vi "Create and configure UDL.vi"(8 "error in":errorcluster, 11 "file path (use dialog)":path) -> (0 "error out":errorcluster, 3 "UDL path":path)   [LabVIEW 2013, in "Database Lib.lvlib"]
uses:
  Database Lib.lvlib
panel:
  out "string":string
  out "cancelled":bool
  out "text":string
  # "Provider=;\nData Source=;\nMode=ReadWrite;\nPersist Security Info=False"
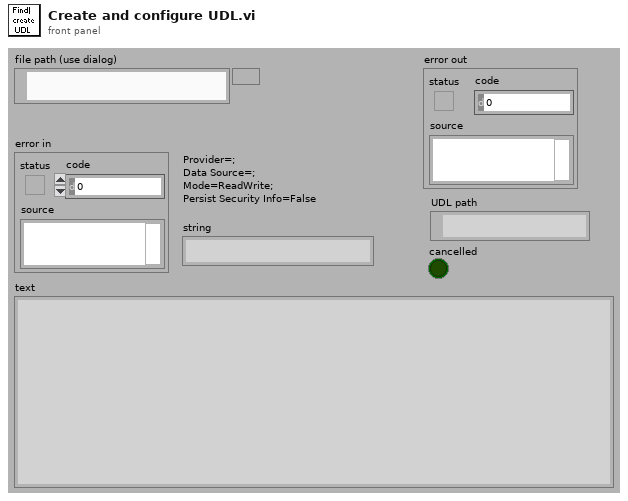
[diagram p1: front panel]
types:
  T1 = enum16{"open", "replace", "create", "open or create", "replace or create", "replace or create with confirmation"}
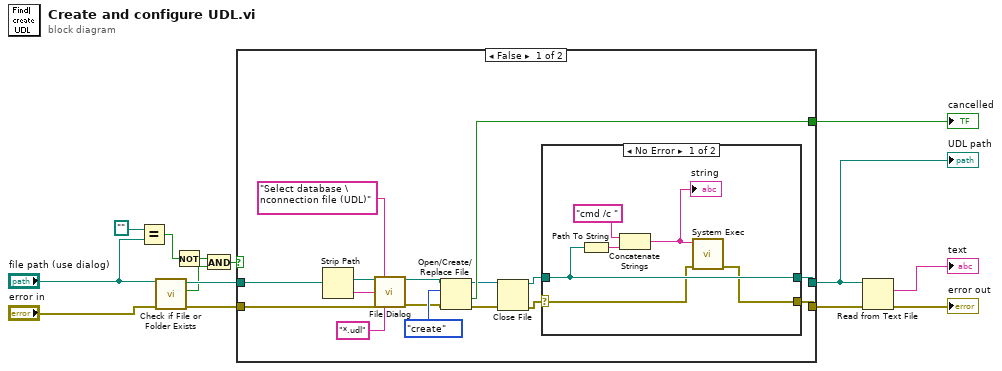
[diagram p0: block diagram]
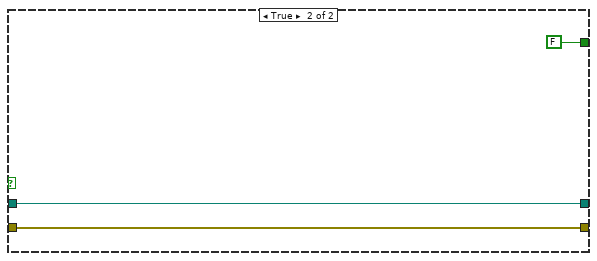
[diagram p3: hidden frame]
diagram:
  n1 = Equal?(x=path "", y="file path (use dialog)") -> (x = y?=w1:bool)
  n2 = call <vilib>:"Check if File or Folder Exists.vi"("error in (no error)"="error in", "path"="file path (use dialog)") -> ("error out"=w10:errorcluster, "file or folder exists?"=w5:bool, "dup path"=w11:path)  [unwired: 7 out]
  n3 = Not(x=w1) -> (.not. x?=w2:bool)
  n4 = And(x=w2, y=w5) -> (x .and. y?=w6:bool)
  n5 = case shown="False" w6 {
    tunnel: w11 -> [w15 w40]
    tunnel: w10 -> [w22 w41]
    tunnel: [w25 w41] -> w9
    tunnel: [w23 w40] -> w7
    tunnel: [w29 FALSE ("cancelled")] -> w8
    frame False {
      n6 = Strip Path(path=w15) -> (stripped path=w17:path, name=w16:string)
      n7 = call "File Dialog"("start path"=w17, "prompt"="Select database \nconnection file (UDL)", "default name"=w16, "error in"=w22, "pattern (all files)"="*.udl") -> ("selected path"=w20:path, "error out"=w21:errorcluster)  [unwired: 2 in, 7 out]
      n8 = Open/Create/Replace File(file path (use dialog)=w20, error in=w21, operation (0:open)=T1."create") -> (refnum out=w27:refnum<file>, cancelled=w29:bool, error out=w28:errorcluster)  [unwired: 3 out]
      n9 = Close File(refnum=w27, error in=w28) -> (path=w24:path, error out=w26:errorcluster)
      n10 = case shown="No Error" w26 {
        selector: w26 -> [w35 w38]
        tunnel: [w34 w38] -> w25
        tunnel: w24 -> [w36 w37]
        tunnel: [w36 w37] -> w23
        frame No Error {
          n11 = Path To String(path=w36) -> (string=w33:string)
          n12 = Concatenate Strings("cmd /c " ("string"), w33) -> (w32:string)
          "string" <- w32
          n13 = call <vilib>:"System Exec.vi"("error in (no error)"=w35, "command line"=w32) -> ("error out"=w34:errorcluster)  [unwired: 4 in, 5 out]
        }
        frame Error {
        }
      }
    }
    frame True {
    }
  }
  "cancelled" <- w8
  "UDL path" <- w7
  n14 = Read from Text File(file (use dialog)=w7, error in=w9) -> (text=→"text":string, error out=→"error out":errorcluster)  [unwired: 4 out]
